vi "Read Stop If Fail.vi"(8 "error in (no error)":errorcluster, 11 "Step in":refnum<class "Step.lvclass">) -> (0 "error out":errorcluster, 2 "Stop If Fail":bool, 3 "Step out":refnum<class "Step.lvclass">)   [LabVIEW 2015, in "Step.lvclass"]
uses:
  Step.lvclass
  Step.lvclass/Step.ctl
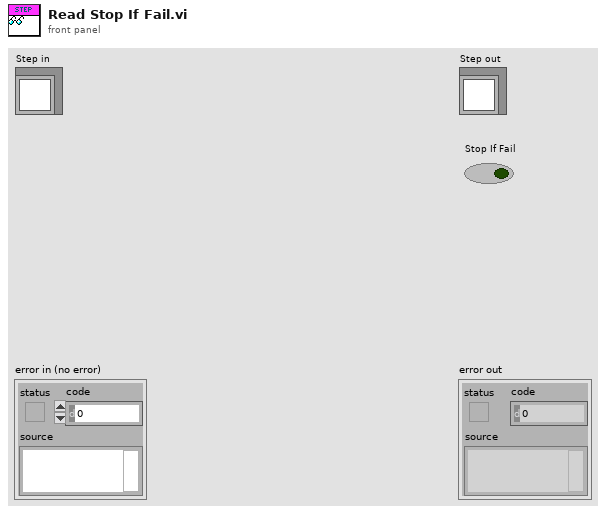
[diagram p1: front panel]
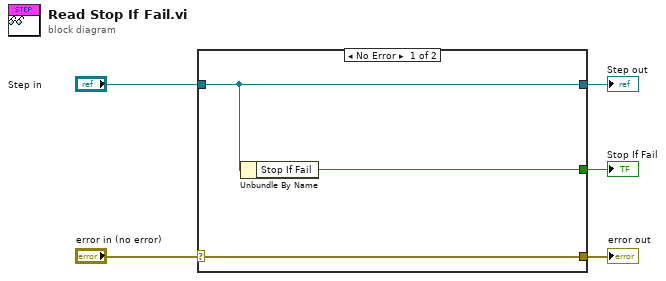
[diagram p0: block diagram]
diagram:
  n1 = case shown="No Error" "error in (no error)" {
    selector: "error in (no error)" -> [w8 w9]
    tunnel: [w8 w9] -> w4
    tunnel: [w7 w10] -> w2
    tunnel: "Step in" -> [w7 w10]
    tunnel: [w6 _] -> w1
    frame No Error {
      n2 = Unbundle By Name(w7) -> ("Stop If Fail"=w6:bool)
    }
    frame Error {
    }
  }
  "error out" <- w4
  "Step out" <- w2
  "Stop If Fail" <- w1
